vi "Untitled 2 (SubVI).vi"(9 "cam0":T1, 10 "cam 0":T1, 11 "MagAnalysis_Online in":refnum<class "MagAnalysis_Online.lvclass">) -> (1 "Cam Cluster out 2":T2, 2 "spec cluster":cluster{"dp [MeV/C]":dbl[], dbl[]}, 3 "z":dbl[][](array[numeric]))   [LabVIEW 2011]
uses:
  shared/OnOffTypeDef.ctl
  lens_TypDEf.ctl
  CamSettingSUB_TypDEf.ctl
  calib_Sub_Typdef.ctl
  ROIInfo_TypDef.ctl
  ScreenCam_TypDEf.ctl
  MagAnalysis_Online.lvclass
  <vilib>/vision/Image Controls.llb/IMAQ Image.ctl
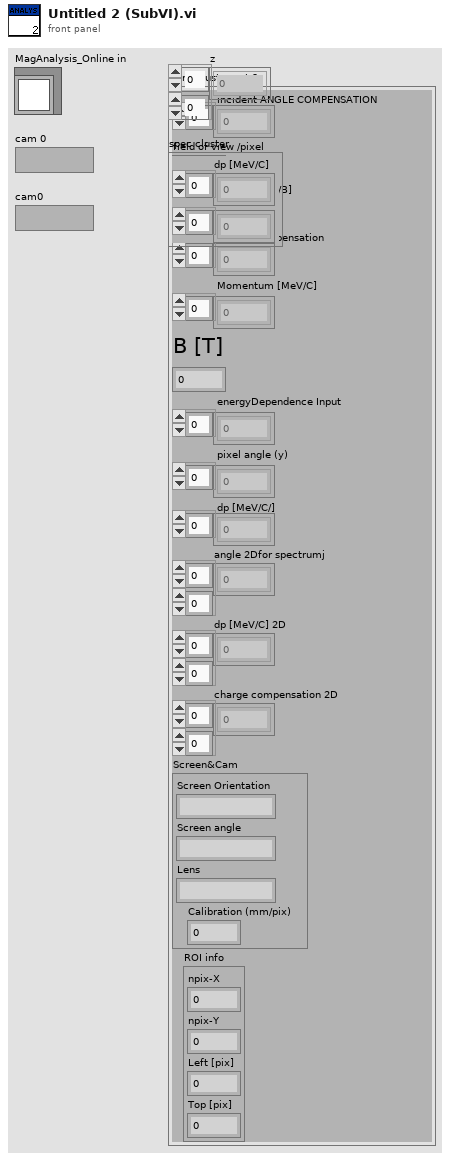
[diagram p1: front panel]
types:
  T1 = typedef "IMAQ Image.ctl" = refnum<image>
  T2 = typedef "calib_Sub_Typdef.ctl" = cluster{"incident ANGLE COMPENSATION":dbl[], "field of view /pixel":dbl, "dp/B [MeV/C/B]":dbl[], "charge compensation":dbl[], "Momentum [MeV/C]":dbl[], "B [T]":dbl, "energyDependence Input":dbl[], "pixel angle (y)":dbl[], "dp [MeV/C/] ":dbl[], "angle 2Dfor spectrumj":dbl[][], "dp [MeV/C] 2D":dbl[][], "charge compensation 2D":dbl[][], "Screen&Cam":T3, "ROI info":T4}
  T3 = typedef "ScreenCam_TypDEf.ctl" = cluster{"Screen Orientation":string, "Screen angle":string, "Lens":string, "Calibration (mm/pix)":dbl}
  T4 = typedef "ROIInfo_TypDef.ctl" = cluster{"npix-X":i32, "npix-Y":i32, "Left [pix]":dbl, "Top [pix]":dbl}
  T5 = typedef "CamSettingSUB_TypDEf.ctl" = cluster{"position":dbl, "Field of view":dbl, "start":dbl, "end":dbl, "center":dbl, "Lens":T6, "Forward":T7, "Spec_Calib_file 2":path, "map":path, "y size":i32}
  T6 = typedef "lens_TypDEf.ctl" = string
  T7 = typedef "OnOffTypeDef.ctl" = enum16{"off", "on"}
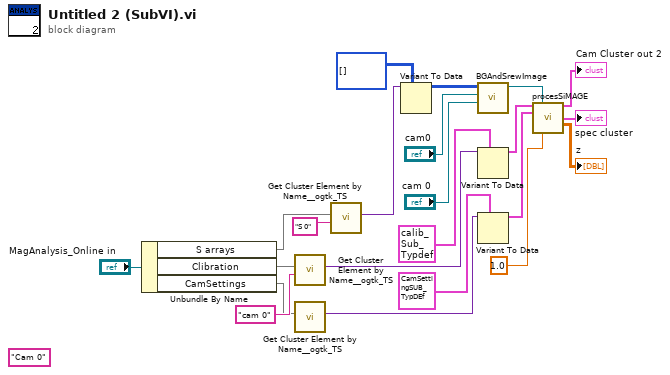
[diagram p0: block diagram]
diagram:
  (unwired) "Cam 0" ("Element Name")
  n1 = Unbundle By Name("MagAnalysis_Online in") -> ("S arrays"=w8, "Clibration"=w18, "CamSettings"=w14)
  n2 = call "Get Cluster Element by Name__ogtk_TS.vi"("Element Name"="cam 0", "Cluster"=w18) -> ("VElement"=w19:variant)  [unwired: 7 in, 2 out]
  n3 = call "Get Cluster Element by Name__ogtk_TS.vi"("Cluster"=w14) -> ("VElement"=w13:variant)  [unwired: 8 in, 2 out]
  n4 = call "Get Cluster Element by Name__ogtk_TS.vi"("Element Name"="S 0", "Cluster"=w8) -> ("VElement"=w10:variant)  [unwired: 7 in, 2 out]
  n5 = Variant To Data(type=i32[][] [] ("S 0"), Variant=w10) -> (data=w12:i32[][])  [unwired: 1 in, 1 out]
  n6 = call "BGAndSrewImage.vi"("BG Image"="cam 0", "Image"="cam0", "S arrays.S 0"=w12) -> ("Image Out"=w1:T1)  [unwired: 6 in, 2 out]
  n7 = Variant To Data(type=T2 {"incident ANGLE COMPENSATION"=[], "field of view /pixel"=0.0, "dp/B [MeV/C/B]"=[], "charge compensation"=[], "Momentum [MeV/C]"=[], "B [T]"=1.0, "energyDependence Input"=[], "pixel angle (y)"=[], "dp [MeV/C/] "=[], "angle 2Dfor spectrumj"=[], "dp [MeV/C] 2D"=[], "charge compensation 2D"=[], "Screen&Cam"={"Screen Orientation"="", "Screen angle"="", "Lens"="", "Calibration (mm/pix)"=0.0}, "ROI info"={"npix-X"=0, "npix-Y"=0, "Left [pix]"=0.0, "Top [pix]"=0.0}} ("cam 0"), Variant=w19) -> (data=w21:T2)  [unwired: 1 in, 1 out]
  n8 = Variant To Data(type=T5 {"position"=0.0, "Field of view"=0.0, "start"=0.0, "end"=0.0, "center"=0.0, "Lens"="f8x06", "Forward"=enum."off", "Spec_Calib_file 2"=path "Y:/100TWdata/ESMCalib/datFwd.txt", "map"=path "Y:/100TWdata/ESMCalib/mapFwd.txt", "y size"=0} ("Cam 0"), Variant=w13) -> (data=w16:T5)  [unwired: 1 in, 1 out]
  n9 = call "procesSiMAGE.vi"("Cam Cluster out"=w21, "Image"=w1, "CamSettings.Cam 0"=w16, "B [T]"=1.0) -> ("Cam Cluster out 2"=→"Cam Cluster out 2":T2, "spec cluster"=→"spec cluster":cluster{"dp [MeV/C]":dbl[], dbl[]}, "z"=→"z":dbl[][])  [unwired: 8 in, 1 out]
